vi "Send RequestShapes Event.vi"(8 "error in (no error)":errorcluster, 10 "Shape Class Filter":string, 11 "Editor Handler in":refnum<class "Image Editor Handler.lvclass">) -> (0 "error out":errorcluster, 2 "Shapes":refnum<data-value>[](array[refnum]), 3 "Editor Handler out":refnum<class "Image Editor Handler.lvclass">)   [LabVIEW 2015, in "LV Image Editor Framework.lvlib" / "Image Editor Handler.lvclass"]
uses:
  Image Editor Handler.lvclass
  Forms/Shape/Shape.lvclass
  Image Editor Handler.lvclass/Image Editor Handler.ctl
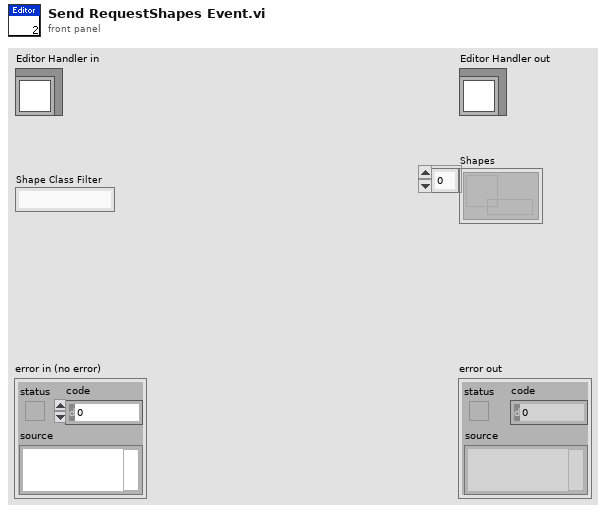
[diagram p1: front panel]
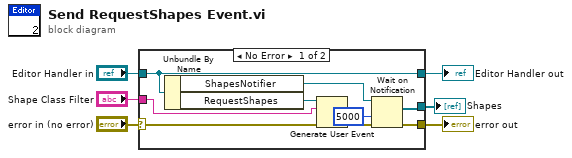
[diagram p0: block diagram]
diagram:
  n1 = case shown="No Error" "error in (no error)" {
    selector: "error in (no error)" -> [w13 w17]
    tunnel: [w10 w17] -> w5
    tunnel: [w15 w16] -> w3
    tunnel: "Editor Handler in" -> [w15 w16]
    tunnel: "Shape Class Filter" -> [w12 _]
    tunnel: [w8 _] -> w1
    frame No Error {
      n2 = Unbundle By Name(w15) -> ("ShapesNotifier"=w9:refnum<notifier>, "RequestShapes"=w14:refnum<user-event>)
      n3 = Generate User Event(user event=w14, event data cluster=w12, error in=w13) -> (error out=w11:errorcluster)  [unwired: 1 in, 1 out]
      n4 = Wait on Notification(notifier=w9, timeout in ms (-1)=5000, error in (no error)=w11) -> (notification=w8:refnum<data-value>[], error out=w10:errorcluster)  [unwired: 1 in, 2 out]
    }
    frame Error {
    }
  }
  "error out" <- w5
  "Editor Handler out" <- w3
  "Shapes" <- w1
